vi "lights_swap.vi"() -> ()   [LabVIEW 2014]
panel:
  out "appended array":sgl[][](array[numeric])
  in  "Array":sgl[][](array[numeric])
  # "This is a hack to swap the first and third tip lights, which are swapped in hardware.  After tip light calibration the triad error is excessive because we are matching the wrong lights when we do the triad error check (and probably our pose is flipped)."
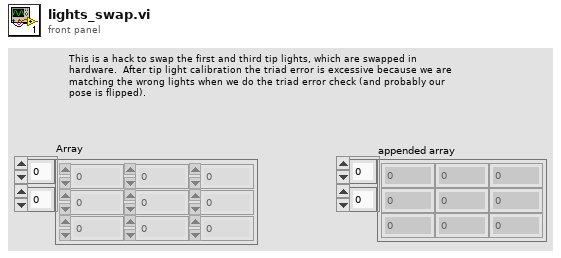
[diagram p1: front panel]
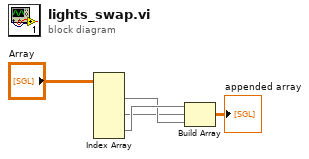
[diagram p0: block diagram]
diagram:
  n1 = Index Array(array="Array") -> (element #1=w3:sgl[], element #2=w2:sgl[], element #3=w4:sgl[])  [unwired: 6 in]
  n2 = Build Array(w4, w2, w3) -> (→"appended array":sgl[][])
